vi "abort.vi"(8 "error in (no error)":errorcluster caption="错误输入（无错误）", 11 "2601B 输入":refnum<class "2601B.lvclass">) -> (0 "error out":errorcluster caption="错误输出", 3 "2601B 输出":refnum<class "2601B.lvclass">)   [LabVIEW 2020, in "2601B.lvclass"]
uses:
  2601B.lvclass
  2601B.lvclass/2601B.ctl
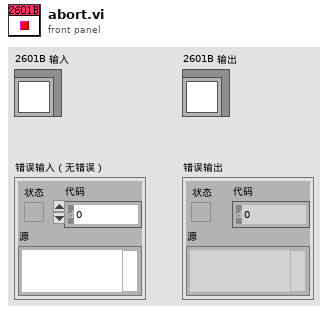
[diagram p1: front panel]
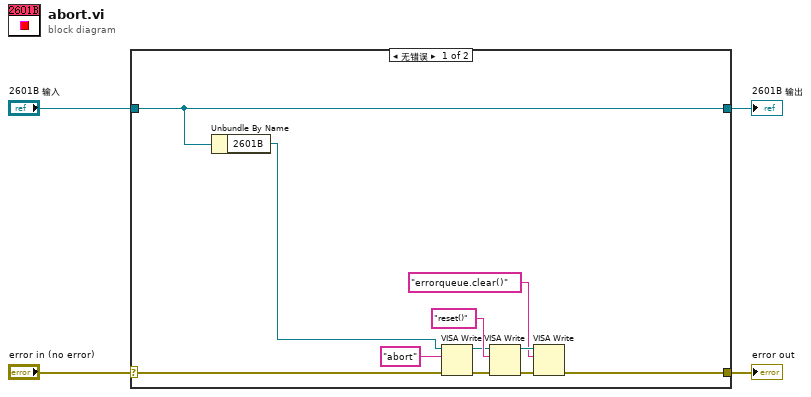
[diagram p0: block diagram]
diagram:
  n1 = case shown="无错误" "error in (no error)" {
    selector: "error in (no error)" -> [w10 w17]
    tunnel: [w7 w17] -> w3
    tunnel: [w15 w16] -> w1
    tunnel: "2601B 输入" -> [w15 w16]
    frame No Error {
      n2 = Unbundle By Name(w15) -> ("2601B"=w9:refnum<visa-resource-name>)
      n3 = VISA Write(VISA resource name=w9, write buffer="abort" ("写入缓冲区"), error in (no error)=w10) -> (VISA resource name out=w13:refnum<visa-resource-name>, error out=w12:errorcluster)  [unwired: 1 out]
      n4 = VISA Write(VISA resource name=w13, write buffer="reset()" ("写入缓冲区"), error in (no error)=w12) -> (VISA resource name out=w6:refnum<visa-resource-name>, error out=w8:errorcluster)  [unwired: 1 out]
      n5 = VISA Write(VISA resource name=w6, write buffer="errorqueue.clear()" ("写入缓冲区"), error in (no error)=w8) -> (error out=w7:errorcluster)  [unwired: 2 out]
    }
    frame Error {
    }
  }
  "error out" <- w3
  "2601B 输出" <- w1
